vi "LIA Example Host Basic.vi"() -> ()   [LabVIEW 2017]
uses:
  lib/host/Public/lock-in settings.ctl
  <vilib>/Analysis/baseanly.llb/Mean (DBL).vi
  <vilib>/FPGAPlugInAG/PXIe-7976R/niLvFpga_Open_PXIe-7976R.vi
  <vilib>/rvi/interface/common/dynamic/niFpgaDynamicAddResources.vi
  <vilib>/FPGAPlugInAG/Dynamic/niLvFpga_Close_Dynamic.vi
  <vilib>/rvi/interface/nirviOpenFPGA/nirviOpenFPGA.xnode
  targets/7976/bitfiles/LIA 7976 5783.lvbitx
  <vilib>/rvi/interface/nirviCloseFPGA/nirviCloseFPGA.xnode
  lib/host/Lock-In Amplifier Example Host.lvlib
  <vilib>/Analysis/NI_AALBase.lvlib
panel:
  out "Waveform Chart":dbl(graph)
  in  "stop":bool
  in  "config":T1
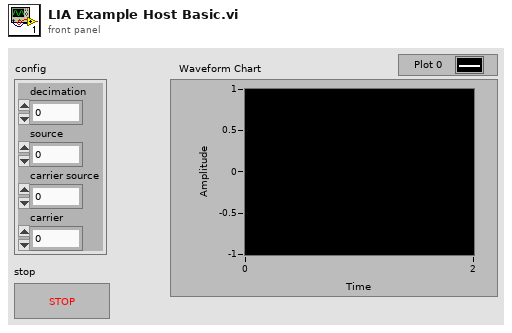
[diagram p1: front panel]
types:
  T1 = typedef "Lock-In Amplifier Example Host.lvlib/lock-in settings.ctl" = cluster{"decimation":i32, "source":i32, "carrier source":i32, "carrier":dbl}
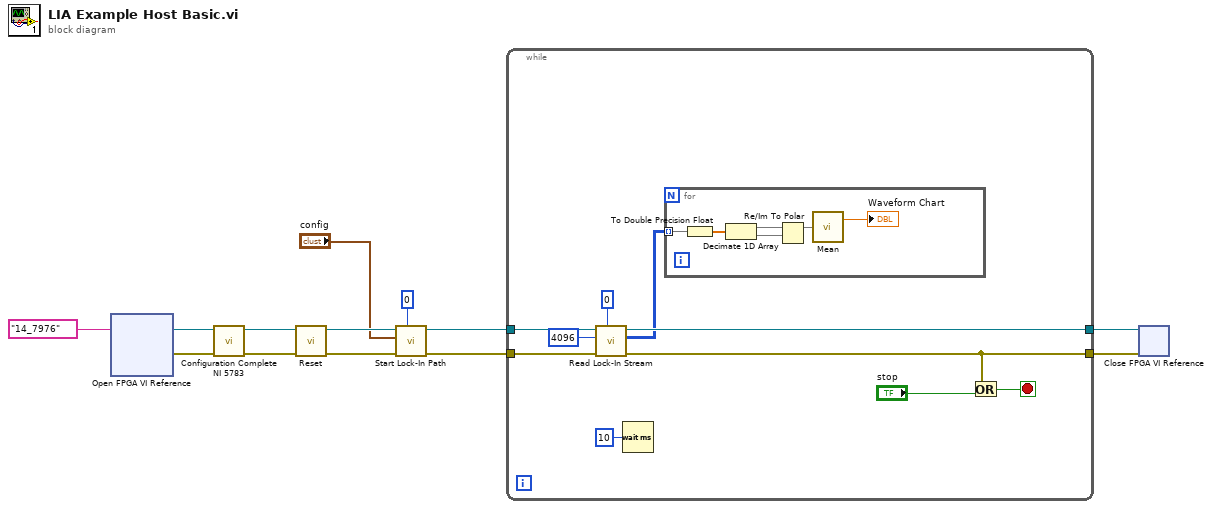
[diagram p0: block diagram]
diagram:
  n1 = xnode "Open FPGA VI Reference"("resource name"=tag "14_7976") -> ("FPGA VI Reference Out"=w6:refnum<k20>, "error out"=w3:errorcluster)  [unwired: 1 in]
  n2 = call "Configuration Complete NI 5783.vi"("error in"=w3, "fpga session in"=w6) -> ("error out"=w4:errorcluster, "fpga session out"=w5:refnum<k20>)  [unwired: 7 in, 1 out]
  n3 = call "Reset.vi"("error in"=w4, "fpga session in"=w5) -> ("error out"=w13:errorcluster, "fpga session out"=w12:refnum<k20>)  [unwired: 8 in]
  n4 = call "Start Lock-In Path.vi"("instance"=0 ("index"), "error in"=w13, "config"="config", "fpga session in"=w12) -> ("error out"=w8:errorcluster, "fpga session out"=w9:refnum<k20>)  [unwired: 6 in]
  n5 = while {
    tunnel: w9 -> [w23]
    tunnel: w8 -> [w22]
    tunnel: [w19] -> w2
    tunnel: [w18] -> w1
    stop <- w17 stop-if-true
    n6 = call "Read Lock-In Stream.vi"("index"=0, "error in"=w22, "elements"=u32 4096, "fpga session in"=w23) -> ("error out"=w18:errorcluster, "unscaled data"=w14:i64[][], "fpga session out"=w19:refnum<k20>)  [unwired: 4 in, 1 out]
    n7 = Wait (ms)(milliseconds to wait=u32 10) -> ()  [unwired: 1 out]
    n8 = for {
      tunnel: w14 -> [w29] mode=indexing
      n9 = To Double Precision Float(number=w29) -> (double precision float=w28:dbl[])
      n10 = Decimate 1D Array(w28) -> (w27:dbl[], w26:dbl[])
      n11 = Re/Im To Polar(2:w26, 3:w27) -> (1:w25:dbl[])  [unwired: 1 out]
      n12 = call-poly <vilib>:"Mean.vi"("X"=w25) -> ("mean"=→"Waveform Chart":dbl)  [unwired: 1 out]
    }
    n13 = Or(x=w18, y="stop") -> (x .or. y?=w17:bool)
  }
  n14 = xnode "Close FPGA VI Reference"("FPGA VI Reference In"=w2, "error in"=w1) -> ()  [unwired: 1 out]
